vi "ActuatorControls.vi"(0 "Boolean in":refnum<vi>, 1 "reference in":refnum<vi>, 2 "Sort  Control":bool, 3 "Reject Control":bool, 5 "reference 3":refnum<vi>, 7 "reference 4":refnum<vi>, 9 "reference 5":refnum<vi>, 12 "Feeder Control":bool, 13 "Belt Control":bool, 14 "Hopper Control":bool) -> (4 "Feeder Light":bool, 6 "Reject Solenoid":bool, 8 "Belt Light":bool, 10 "Sort Solenoid":bool, 15 "Hopper  Actuator":bool)   [LabVIEW 2016]
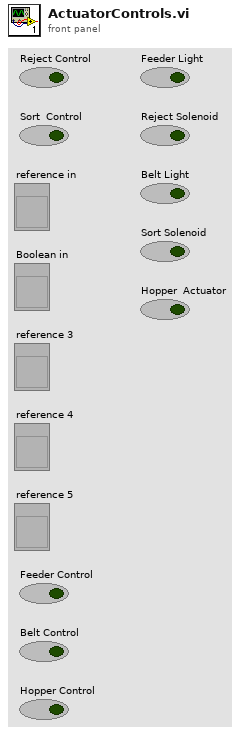
[diagram p1: front panel]
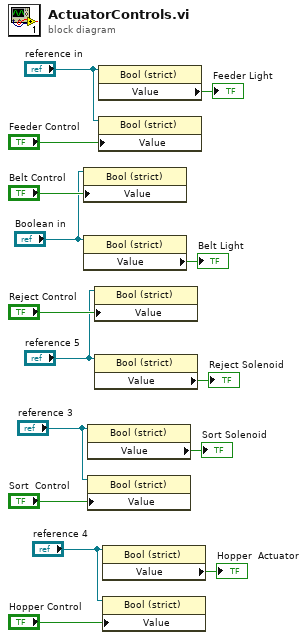
[diagram p0: block diagram]
diagram:
  n1 = property class="Bool (strict)"(reference="Boolean in", "Value"="Belt Control") -> ()  [unwired: 1 in, 2 out]
  n2 = property class="Bool (strict)"(reference="Boolean in") -> ("Value"=→"Belt Light":bool)  [unwired: 1 in, 2 out]
  n3 = property class="Bool (strict)"(reference="reference 3") -> ("Value"=→"Sort Solenoid":bool)  [unwired: 1 in, 2 out]
  n4 = property class="Bool (strict)"(reference="reference 3", "Value"="Sort  Control") -> ()  [unwired: 1 in, 2 out]
  n5 = property class="Bool (strict)"(reference="reference 5", "Value"="Reject Control") -> ()  [unwired: 1 in, 2 out]
  n6 = property class="Bool (strict)"(reference="reference 5") -> ("Value"=→"Reject Solenoid":bool)  [unwired: 1 in, 2 out]
  n7 = property class="Bool (strict)"(reference="reference in") -> ("Value"=→"Feeder Light":bool)  [unwired: 1 in, 2 out]
  n8 = property class="Bool (strict)"(reference="reference in", "Value"="Feeder Control") -> ()  [unwired: 1 in, 2 out]
  n9 = property class="Bool (strict)"(reference="reference 4") -> ("Value"=→"Hopper  Actuator":bool)  [unwired: 1 in, 2 out]
  n10 = property class="Bool (strict)"(reference="reference 4", "Value"="Hopper Control") -> ()  [unwired: 1 in, 2 out]
